vi "Binary Search on One Hot Encoded Number (U64)_no pipeline.vi"(10 "One Hot encoded Number":u64 format="%064b") -> (2 "Binary Number":u8)   [LabVIEW 2011]
panel:
  out "Leading One Position":bool[](array[boolean])
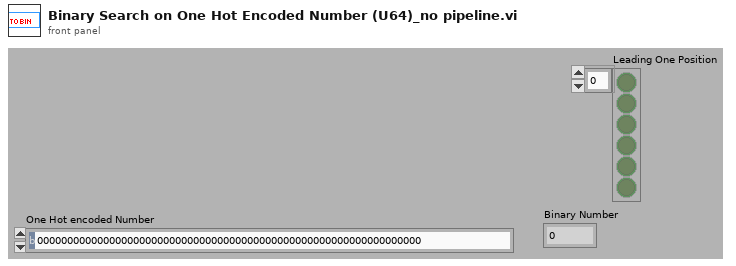
[diagram p1: front panel]
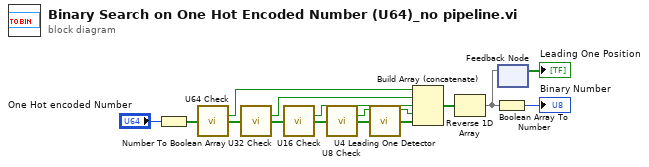
[diagram p0: block diagram]
diagram:
  n1 = Number To Boolean Array(number="One Hot encoded Number") -> (Boolean array=w2:bool[])
  n2 = call <userlib>:"U64 Check.vi"("64--bit array"=w2) -> ("Lower Half has one?"=w8:bool, "Half with one?"=w15:bool[])  [unwired: 13 in]
  n3 = call <userlib>:"U32 Check.vi"("32-bit array"=w15) -> ("Lower Half has one?"=w9:bool, "Half with one?"=w1:bool[])  [unwired: 13 in]
  n4 = call <userlib>:"U16 Check.vi"("16-bit array"=w1) -> ("Lower Half has one?"=w10:bool, "Half with one?"=w14:bool[])  [unwired: 13 in]
  n5 = call <userlib>:"U8 Check.vi"("8-bit array"=w14) -> ("Lower Half has one?"=w11:bool, "Half with one?"=w13:bool[])  [unwired: 13 in]
  n6 = call <userlib>:"U4 Leading One Detector.vi"("4-Bit Array"=w13) -> ("Leading One Position"=w12:bool[])  [unwired: 14 in]
  n7 = Build Array (concatenate)(w8, w9, w10, w11, w12) -> (w7:bool[])
  n8 = Reverse 1D Array(array=w7) -> (reversed array=w4:bool[])
  n9 = Boolean Array To Number(Boolean array=w4) -> (number=→"Binary Number":u8)
  n10 = feedback #1() -> (→"Leading One Position":bool[])  [unwired: 1 in]
  n11 = feedback-in #1(w4) -> ()
